vi "Get Log Path v2.vi"(3 "Log Dir Name":string="Stim Logs") -> (1 "Log Path":path)   [LabVIEW 2019]
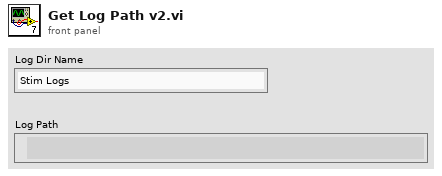
[diagram p1: front panel]
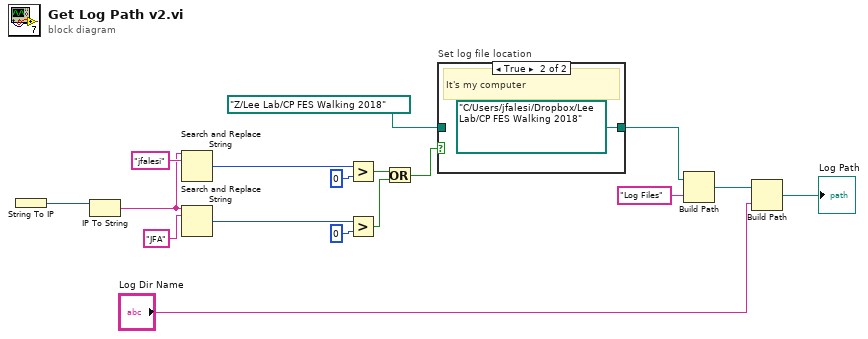
[diagram p0: block diagram]
diagram:
  n1 = String To IP() -> (0:w9:u32)  [unwired: 1 in]
  n2 = IP To String(2:w9) -> (0:w6:string)  [unwired: 1 in]
  n3 = Search and Replace String(input string=w6, search string="jfalesi") -> (number of replacements=w11:i32)  [unwired: 6 in, 3 out]
  n4 = Search and Replace String(input string=w6, search string="JFA") -> (number of replacements=w4:i32)  [unwired: 6 in, 3 out]
  n5 = Greater?(x=w11, y=0) -> (0:w3:bool)
  n6 = Greater?(x=w4, y=0) -> (0:w2:bool)
  n7 = Or(x=w3, y=w2) -> (x .or. y?=w1:bool)
  n8 = case "Set log file location" shown="True" w1 {
    tunnel: [w18 path "C:/Users/jfalesi/Dropbox/Lee Lab/CP FES Walking 2018" ("Stim Log Path")] -> w14
    tunnel: path "Z:/Lee Lab/CP FES Walking 2018" ("Base Data Path") -> [w18 _]
    frame False {
      # "It's the lab computer"
    }
    frame True {
      # "It's my computer"
    }
  }
  n9 = Build Path(base path=w14, name or relative path="Log Files") -> (appended path=w15:path)
  n10 = Build Path(base path=w15, name or relative path="Log Dir Name") -> (appended path=→"Log Path":path)
